vi "Check TestStand.vi"(8 "error in (no error)":errorcluster) -> (0 "error out":errorcluster, 3 "TestStand Check Results":T1)   [LabVIEW 2026, in "Readines Service.lvclass"]
uses:
  Readines Service.lvclass
  Readines Service.lvclass/Readines Service.ctl
  Adapters/TestStand/TestStand Adapter/TestStand Adapter.lvclass
  Typedefs/enums/Readiness State Enum.ctl
  Typedefs/clusters/Readiness Check Result.ctl
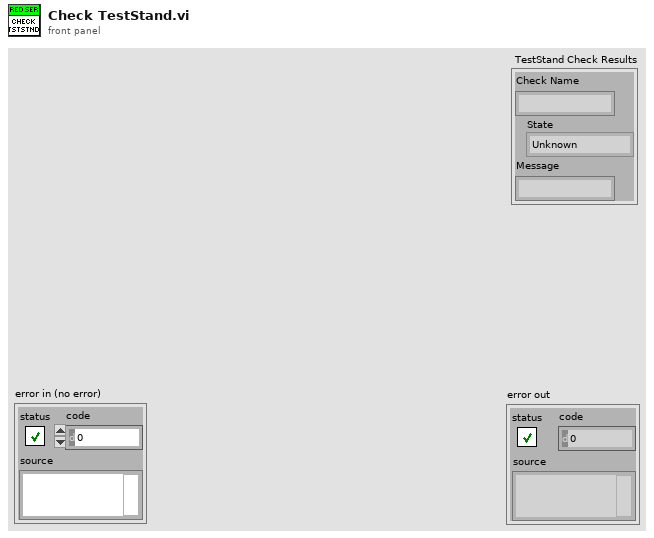
[diagram p1: front panel]
types:
  T1 = typedef "Readiness Check Result.ctl" = cluster{"Check Name":string, "State":T2, "Message":string}
  T2 = typedef "Readiness State Enum.ctl" = enum16{"Unknown", "Ready", "Warning", "NotReady"}
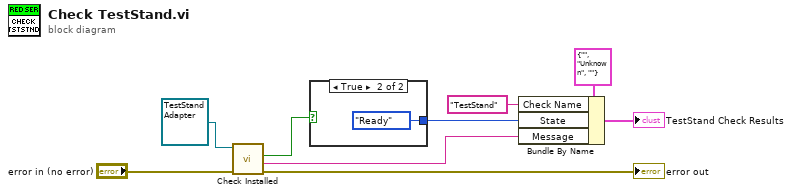
[diagram p0: block diagram]
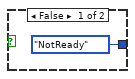
[diagram p2: hidden frame]
diagram:
  n1 = call-dynamic "Check Installed.vi"("error in (no error)"="error in (no error)", "TestStand Adapter in"=refnum<class "TestStand Adapter.lvclass"> refnum ("TestStand Adapter.lvclass")) -> ("error out"=→"error out":errorcluster, "Version"=w1:string, "Installed?"=w3:bool)  [unwired: 6 in, 1 out]
  n2 = case shown="True" w3 {
    tunnel: [Readiness_State_Enum."NotReady" ("State") Readiness_State_Enum."Ready" ("State")] -> w2
    frame False {
    }
    frame True {
    }
  }
  n3 = Bundle By Name(cluster=T1 {"Check Name"="", "State"=enum."Unknown", "Message"=""} ("Readiness Check Result"), "Check Name"="TestStand", "State"=w2, "Message"=w1) -> (→"TestStand Check Results":T1)
